vi "Query Slit Position.vi"(7 "Mono System # (0)":T2, 8 "error in (no error)":errorcluster, 10 "Slit (Front/Axial Entrance)":T1, 11 "VISA resource name":refnum<visa-resource-name>) -> (0 "error out":errorcluster, 1 "Slit Position":dbl[unit], 3 "VISA resource name out":refnum<visa-resource-name>)   [LabVIEW 2009, in "JY-SPEX-TRIAX.lvlib"]
doc: "Queries the current step position of the chosen slit. May be read while the slits are moving."
uses:
  JY-SPEX-TRIAX.lvlib
  controls.llb/Monochromator System Number.ctl
  controls.llb/Slits.ctl
  Spectrometer Config.vi
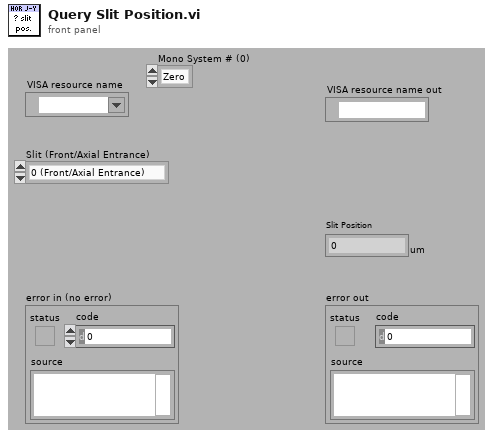
[diagram p1: front panel]
types:
  T1 = typedef "JY-SPEX-TRIAX.lvlib/Slits.ctl" = enum16{"0 (Front/Axial Entrance)", "1 (Side/Lateral Entrance)", "2 (Front/Axial Exit)", "3 (Side/Lateral Exit)"}
  T2 = typedef "JY-SPEX-TRIAX.lvlib/Monochromator System Number.ctl" = enum16{"Zero", "One"}
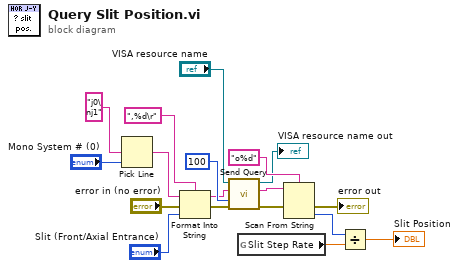
[diagram p0: block diagram]
diagram:
  n1 = Pick Line(multi-line string="j0\nj1", line index="Mono System # (0)") -> (output string=w9:string)  [unwired: 1 out]
  n2 = Format Into String(format string=",%d\r", initial string=w9, error in="error in (no error)", "Slit (Front/Axial Entrance)") -> (resulting string=w4:string, error out=w5:errorcluster)
  n3 = call "Send Query.vi"("error in (no error)"=w5, "byte count"=u32 100, "write buffer"=w4, "VISA resource name"="VISA resource name") -> ("error out"=w12:errorcluster, "read buffer"=w14:string, "VISA resource name out"=→"VISA resource name out":refnum<visa-resource-name>)  [unwired: 5 out]
  n4 = global read "Spectrometer Config.vi" "Slit Step Rate"() -> (w3:dbl[unit])
  n5 = Scan From String(format string="o%d", input string=w14, error in=w12) -> (error out=→"error out":errorcluster, output 1=w2:i32)  [unwired: 1 in, 3 out]
  n6 = Divide(x=w2, y=w3) -> (x/y=→"Slit Position":dbl[unit])
